vi "Graphics-Wavelength to RGB.vi"(7 "Wavelength (nm)":dbl) -> (8 "Color":u32(colorbox))   [LabVIEW 2015]
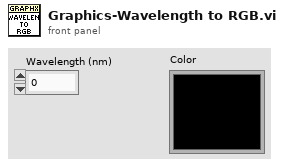
[diagram p1: front panel]
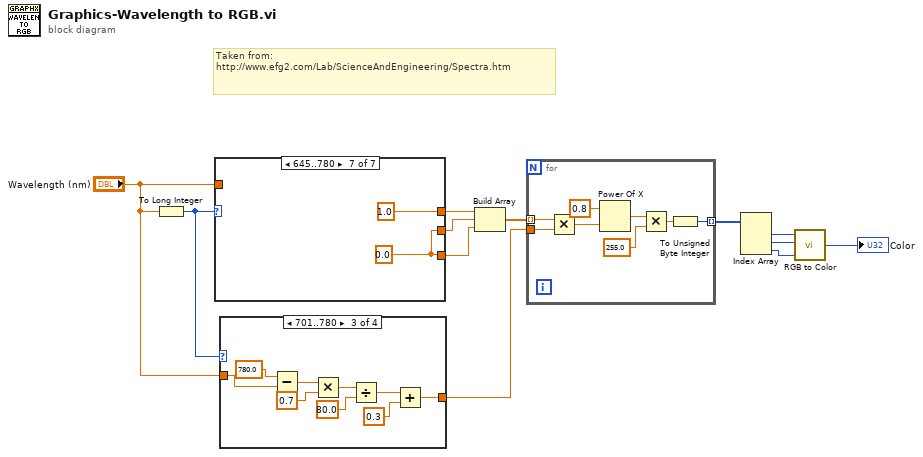
[diagram p0: block diagram]
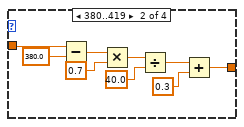
[diagram p3: hidden frame]
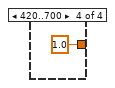
[diagram p4: hidden frame]
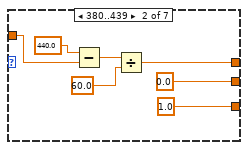
[diagram p6: hidden frame]
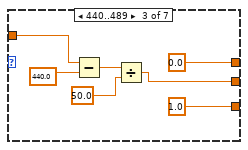
[diagram p7: hidden frame]
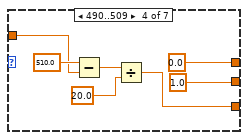
[diagram p8: hidden frame]
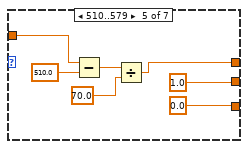
[diagram p9: hidden frame]
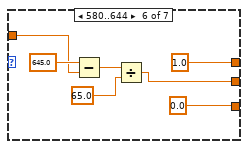
[diagram p10: hidden frame]
diagram:
  # "Taken from:\nhttp://www.efg2.com/Lab/ScienceAndEngineering/Spectra.htm"
  n1 = To Long Integer(number="Wavelength (nm)") -> (32bit integer=w12:i32)
  n2 = case shown="645..780" w12 {
    tunnel: "Wavelength (nm)" -> [_ w16 w23 w30 w37 w44 _]
    tunnel: [_ w15 0.0 0.0 w34 1.0 1.0] -> w10
    tunnel: [_ 0.0 w22 1.0 1.0 w41 w48] -> w9
    tunnel: [_ 1.0 1.0 w27 0.0 0.0 w48] -> w8
    frame 0, Default {
    }
    frame 380..439 {
      n3 = Subtract(x=440.0 ("y"), y=w16) -> (x-y=w18:dbl)
      n4 = Divide(x=w18, y=60.0) -> (x/y=w15:dbl)
    }
    frame 440..489 {
      n5 = Subtract(x=w23, y=440.0) -> (x-y=w25:dbl)
      n6 = Divide(x=w25, y=50.0) -> (x/y=w22:dbl)
    }
    frame 490..509 {
      n7 = Subtract(x=510.0 ("y"), y=w30) -> (x-y=w32:dbl)
      n8 = Divide(x=w32, y=20.0) -> (x/y=w27:dbl)
    }
    frame 510..579 {
      n9 = Subtract(x=w37, y=510.0) -> (x-y=w39:dbl)
      n10 = Divide(x=w39, y=70.0) -> (x/y=w34:dbl)
    }
    frame 580..644 {
      n11 = Subtract(x=645.0 ("y"), y=w44) -> (x-y=w46:dbl)
      n12 = Divide(x=w46, y=65.0) -> (x/y=w41:dbl)
    }
    frame 645..780 {
      w48 = 0.0
    }
  }
  n13 = case shown="701..780" w12 {
    tunnel: "Wavelength (nm)" -> [_ w58 w67 _]
    tunnel: [_ w50 w59 1.0] -> w6
    frame 0, Default {
    }
    frame 380..419 {
      n14 = Subtract(x=w58, y=380.0) -> (x-y=w56:dbl)
      n15 = Multiply(x=w56, y=0.7) -> (x*y=w54:dbl)
      n16 = Divide(x=w54, y=40.0) -> (x/y=w52:dbl)
      n17 = Add(x=w52, y=0.3) -> (x+y=w50:dbl)
    }
    frame 701..780 {
      n18 = Subtract(x=780.0 ("y"), y=w67) -> (x-y=w65:dbl)
      n19 = Multiply(x=w65, y=0.7) -> (x*y=w63:dbl)
      n20 = Divide(x=w63, y=80.0) -> (x/y=w61:dbl)
      n21 = Add(x=w61, y=0.3) -> (x+y=w59:dbl)
    }
    frame 420..700 {
    }
  }
  n22 = Build Array(w10, w9, w8) -> (w7:dbl[])
  n23 = for {
    tunnel: w7 -> [w76] mode=indexing
    tunnel: w6 -> [w75]
    tunnel: [w71] -> w5 mode=indexing
    n24 = Multiply(x=w76, y=w75) -> (x*y=w74:dbl)
    n25 = Power Of X(1:w74, 2:0.8 ("y")) -> (0:w72:dbl)
    n26 = Multiply(x=w72, y=255.0) -> (x*y=w70:dbl)
    n27 = To Unsigned Byte Integer(number=w70) -> (unsigned 8bit integer=w71:u8)
  }
  n28 = Index Array(array=w5) -> (element #1=w4:u8, element #2=w3:u8, element #3=w2:u8)  [unwired: 3 in]
  n29 = call <vilib>:"RGB to Color.vi"("B"=w2, "G"=w3, "R"=w4) -> ("Color"=→"Color":u32)
